vi "Score Macro.vi"   [LabVIEW 2018]
types:
  T1 = typedef "Command Status Info.ctl" = cluster{"Name":string, "Status":T2, "notifier out":T3}
  T2 = typedef "Completion Status.ctl" = enum16{"Successful", "Aborted", "Incomplete"}
  T3 = typedef "Completion Notifier.ctl" = refnum<notifier>
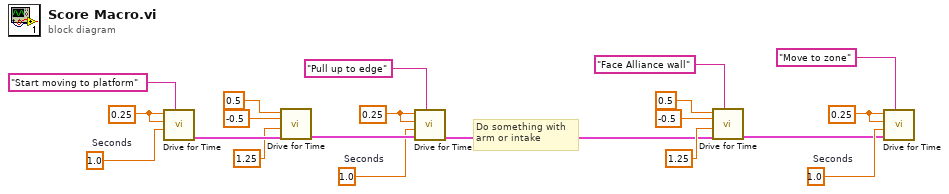
[diagram p0: block diagram]
diagram:
  w8 = 1.0  # Seconds
  w7 = 0.25
  w12 = 1.0  # Seconds
  w14 = 0.25
  w19 = 1.0  # Seconds
  w20 = 0.25
  # "Do something with\narm or intake"
  n1 = call "Drive for Time.vi"("Description"="Start moving to platform", "Seconds"=w19, "Right Speed"=w20, "Left Speed"=w20) -> ("Command Info Out"=w18:T1)  [unwired: 6 in, 1 out]
  n2 = call "Drive for Time.vi"("Command Info In"=w18, "Seconds"=1.25, "Right Speed"=-0.5, "Left Speed"=0.5) -> ("Command Info Out"=w13:T1)  [unwired: 6 in, 1 out]
  n3 = call "Drive for Time.vi"("Description"="Pull up to edge", "Command Info In"=w13, "Seconds"=w12, "Right Speed"=w14, "Left Speed"=w14) -> ("Command Info Out"=w5:T1)  [unwired: 5 in, 1 out]
  n4 = call "Drive for Time.vi"("Description"="Face Alliance wall", "Command Info In"=w5, "Seconds"=1.25, "Right Speed"=-0.5, "Left Speed"=0.5) -> ("Command Info Out"=w6:T1)  [unwired: 5 in, 1 out]
  n5 = call "Drive for Time.vi"("Description"="Move to zone", "Command Info In"=w6, "Seconds"=w8, "Right Speed"=w7, "Left Speed"=w7) -> ()  [unwired: 5 in, 2 out]
